vi "EuniceF_Lab4Labview.vi"() -> ()   [LabVIEW 2025]
panel:
  out "Offset":dbl(slide) scale=0.0..10.0
  out "Weight":dbl(knob) scale=0.0..10.0
  in  "Tare":bool
  out "Load cell Signal, mV":dbl(slide) scale=0.0..10.0 scale format="%1.3g"
  out "Vscc, V":dbl(slide) scale=0.0..10.0 scale format="%1.3g"
  out "AtoD":i16
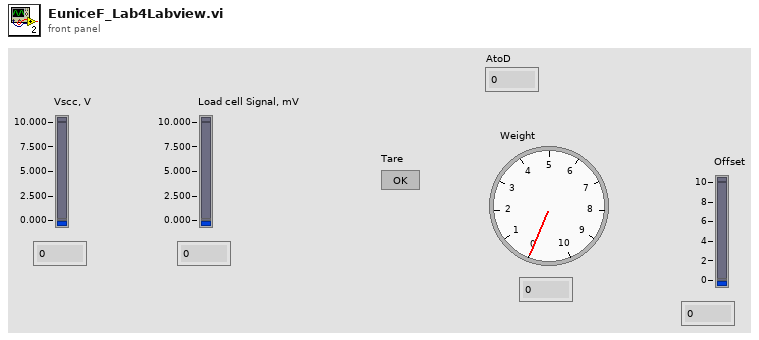
[diagram p1: front panel]
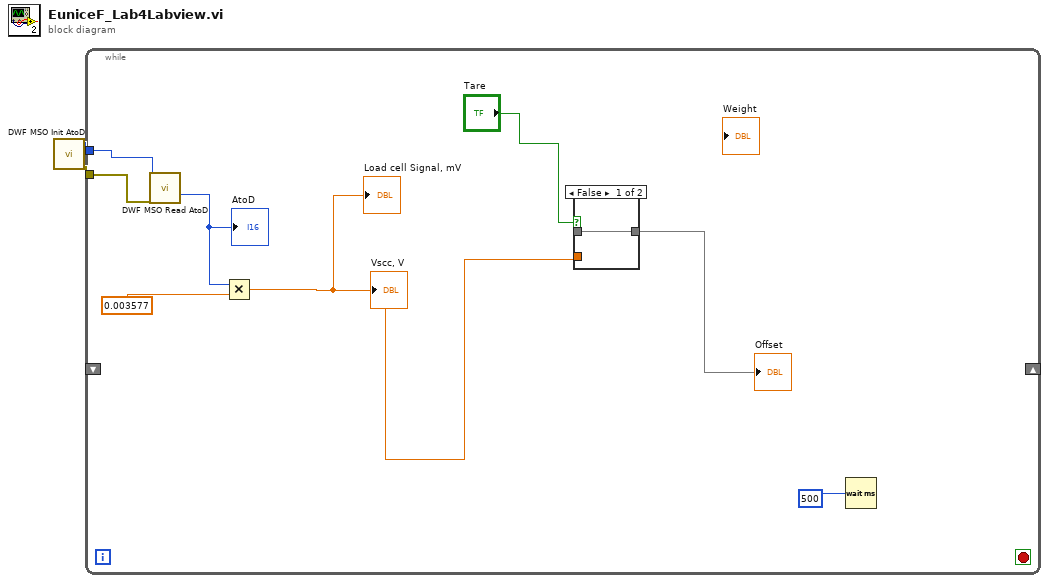
[diagram p0: block diagram]
diagram:
  n1 = call "DWF MSO Init AtoD.vi"() -> ("Error Out"=w1:errorcluster, "Instrument Handle Out"=w2:i32)  [unwired: 10 in]
  n2 = while {
    tunnel: w2 -> [w11]
    tunnel: w1 -> [w10]
    shift-right: _ -> [w5]
    shift-left: _ -> [w3]
    stop <- _ stop-if-true
    n3 = call "DWF MSO Read AtoD.vi"("Instrument Handle In AtoD"=w11, "Error In"=w10) -> ("AtoD"=w9:i16)  [unwired: 12 in, 1 out]
    "AtoD" <- w9
    n4 = Multiply(x=w9, y=0.003577) -> (x*y=w6:dbl)
    "Vscc, V" <- w6
    "Load cell Signal, mV" <- w6
    n5 = case shown="False" "Tare" {
      tunnel: [w14 w15] -> w7
      tunnel: [w14 w15] -> w4
      tunnel: w6 -> [_ _]
      frame False {
      }
      frame True {
      }
    }
    "Offset" <- w7
    n6 = Wait (ms)(milliseconds to wait=u32 500) -> ()  [unwired: 1 out]
  }
